vi "Waveform to XY Graph.vi"(7 "Measure Load Current":T1) -> (8 "Scope Waveform":cluster{dbl[], dbl[]})   [LabVIEW 2020, in "LDO Load Transient.lvlib"]
uses:
  LDO Load Transient.lvlib
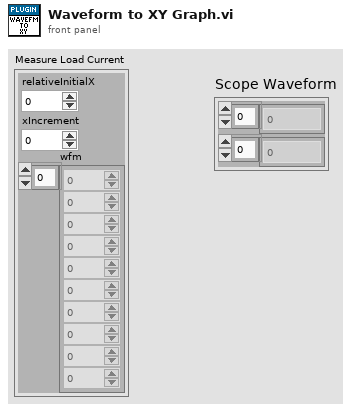
[diagram p1: front panel]
types:
  T1 = cluster{"relativeInitialX":dbl, "xIncrement":dbl, "wfm":dbl[]}
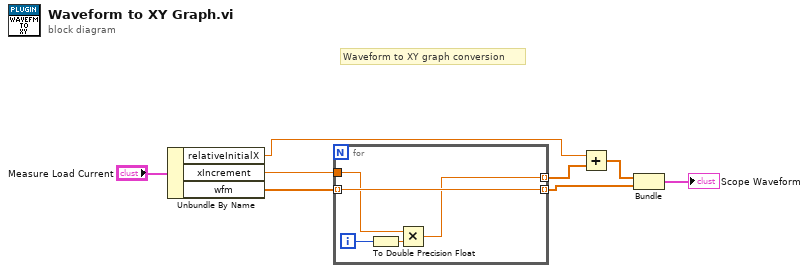
[diagram p0: block diagram]
diagram:
  # "Waveform to XY graph conversion"
  n1 = Unbundle By Name("Measure Load Current") -> ("relativeInitialX"=w3:dbl, "xIncrement"=w6:dbl, "wfm"=w8:dbl[])
  n2 = for {
    tunnel: w6 -> [w9]
    tunnel: [w13] -> w7 mode=indexing
    tunnel: [w10] -> w2 mode=indexing
    tunnel: w8 -> [w13] mode=indexing
    i -> [w12]
    n3 = To Double Precision Float(number=w12) -> (double precision float=w11:dbl)
    n4 = Multiply(x=w9, y=w11) -> (x*y=w10:dbl)
  }
  n5 = Add(x=w3, y=w2) -> (x+y=w1:dbl[])
  n6 = Bundle(w1, w7) -> (→"Scope Waveform":cluster{dbl[], dbl[]})  [unwired: 1 in]
